vi "Get Label.vi"(8 "error in (no error)":errorcluster, 11 "Motor Configuration in":refnum<class "Motor Configuration.lvclass">) -> (0 "error out":errorcluster, 2 "Label":string, 3 "Motor Configuration out":refnum<class "Motor Configuration.lvclass">)   [LabVIEW 2016, in "Hardware.lvlib" / "Motor.lvlib" / "Motor Configuration.lvclass"]
uses:
  <userlib>/Common Components/Hardware/Motor/Motor Config/Motor Configuration.lvclass
  <userlib>/Common Components/Hardware/Motor/Motor Config/Motor Configuration.lvclass/Motor Configuration.ctl
  <userlib>/Common Components/Hardware/Abstract Hardware/Hardware.lvclass/Hardware.ctl
  <userlib>/Common Components/Hardware/Abstract Hardware/Read Label.vi
  <userlib>/Common Components/Hardware/Motor/Motor/Motor.lvclass
  C:/Program Files (x86)/National Instruments/LabVIEW 2016/user.lib/Common Components/Hardware/Abstract Hardware/Hardware.lvclass
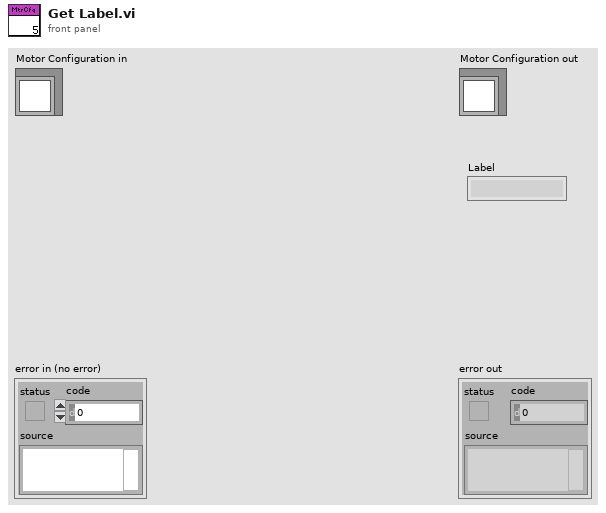
[diagram p1: front panel]
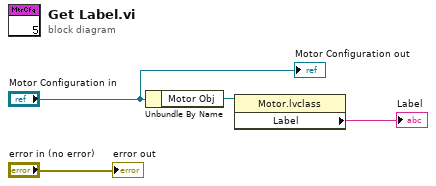
[diagram p0: block diagram]
diagram:
  n1 = Unbundle By Name("Motor Configuration in") -> ("Motor Obj"=w2:refnum<class "Motor.lvclass">)
  n2 = property class="Motor.lvclass"(reference=w2) -> ("Label"=→"Label":string)  [unwired: 1 in, 2 out]
  "error out" <- "error in (no error)"
  "Motor Configuration out" <- "Motor Configuration in"
